vi "old_HWGlobalsToObject.vi"(7 "Select Layout":refnum<vi>, 8 "error in (no error)":errorcluster, 10 "Novatech Channel":T1, 11 "Novatech in":refnum<class "Novatech.lvclass">) -> (0 "error out":errorcluster, 3 "Novatech out":refnum<class "Novatech.lvclass">)   [LabVIEW 2013, in "Novatech.lvclass"]
uses:
  Novatech.lvclass
  Novatech.lvclass/Novatech.ctl
panel:
  # "Why is SetList Display 2d boolean array? The DDS, NI cards are 1d.\nAre layouts stored by row or by column?"
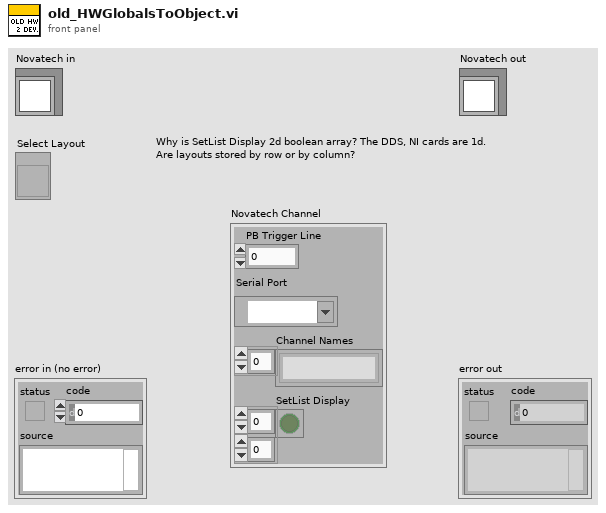
[diagram p1: front panel]
types:
  T1 = cluster{"PB Trigger Line":u16, "Serial Port":refnum<visa-resource-name>, "Channel Names":string[], "SetList Display":bool[][]}
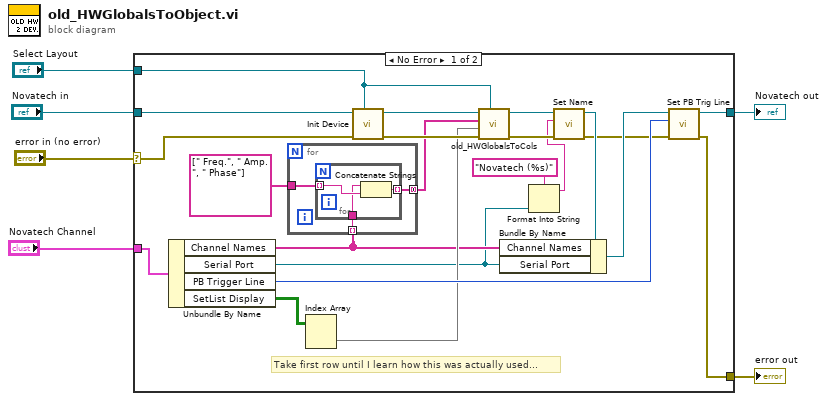
[diagram p0: block diagram]
diagram:
  n1 = case shown="No Error" "error in (no error)" {
    selector: "error in (no error)" -> [w22 w36]
    tunnel: [w24 w36] -> w5
    tunnel: [w25 w35] -> w3
    tunnel: "Novatech in" -> [w23 w35]
    tunnel: "Novatech Channel" -> [w28 _]
    tunnel: "Select Layout" -> [w19 _]
    frame No Error {
      # "Take first row until I learn how this was actually used..."
      n2 = Unbundle By Name(w28) -> ("Channel Names"=w15:string[], "Serial Port"=w8:refnum<visa-resource-name>, "PB Trigger Line"=w26:u16, "SetList Display"=w18:bool[][])
      n3 = for {
        tunnel: string[] [" Freq.", " Amp.", " Phase"] -> [w31]
        tunnel: w15 -> [w30] mode=indexing
        tunnel: [w29] -> w14 mode=concatenating
        n4 = for {
          tunnel: w31 -> [w34] mode=indexing
          tunnel: w30 -> [w33]
          tunnel: [w32] -> w29 mode=indexing
          n5 = Concatenate Strings(w33, w34) -> (w32:string)
        }
      }
      n6 = Index Array(array=w18) -> (element=w17:bool[])  [unwired: 2 in]
      n7 = call-dynamic "Init Device.vi"("Layout Ref"=w19, "error in (no error)"=w22, "Novatech in"=w23) -> ("error out"=w20:errorcluster, "Novatech out"=w21:refnum<class "Novatech.lvclass">)  [unwired: 7 in]
      n8 = call-dynamic "old_HWGlobalsToCols.vi"("Select Layout"=w19, "error in (no error)"=w20, "SetList Display"=w17, "Column Names"=w14, "Device in"=w21) -> ("error out"=w11:errorcluster, "Device out"=w13:refnum<class "Novatech.lvclass">)  [unwired: 5 in]
      n9 = Format Into String(format string="Novatech (%s)", w8) -> (resulting string=w7:string)  [unwired: 2 in, 1 out]
      n10 = call-dynamic "Set Name.vi"("error in (no error)"=w11, "Name"=w7, "Device in"=w13) -> ("error out"=w10:errorcluster, "Device out"=w12:refnum<class "Novatech.lvclass">)  [unwired: 7 in]
      n11 = Bundle By Name(cluster=w12, "Channel Names"=w15, "Serial Port"=w8) -> (w27:refnum<class "Novatech.lvclass">)
      n12 = call-dynamic "Set PB Trig Line.vi"("error in (no error)"=w10, "PB Trigger Line"=w26, "Device in"=w27) -> ("error out"=w24:errorcluster, "Device out"=w25:refnum<class "Novatech.lvclass">)  [unwired: 7 in]
    }
    frame Error {
    }
  }
  "error out" <- w5
  "Novatech out" <- w3
